vi "SPI_WRITE.vi"(0 "size(s) IN":i32, 1 "Data":u8) -> (6 "size(s)":i32, 7 "SDA":bool[](array[boolean]), 8 "SCL":bool[](array[boolean]), 9 "PFIWE":bool[](array[boolean]), 10 "ACK":i32)   [LabVIEW 2018]
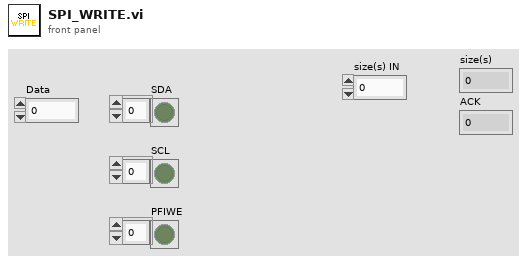
[diagram p1: front panel]
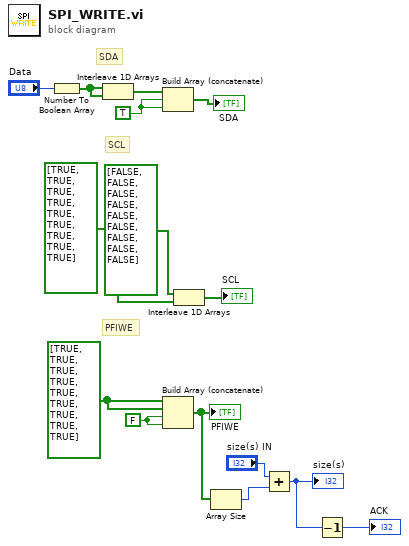
[diagram p0: block diagram]
diagram:
  w15 = FALSE
  w12 = TRUE
  w9 = bool[] [TRUE, TRUE, TRUE, TRUE, TRUE, TRUE, TRUE, TRUE, TRUE]
  # "PFIWE"
  # "SCL"
  # "SDA"
  n1 = Number To Boolean Array(number="Data") -> (Boolean array=w6:bool[])
  n2 = Interleave 1D Arrays(w6, w6) -> (w7:bool[])
  n3 = Build Array (concatenate)(w7, w12, w12) -> (→"SDA":bool[])
  n4 = Build Array (concatenate)(w9, w9, w15, w15) -> (w5:bool[])
  "PFIWE" <- w5
  n5 = Interleave 1D Arrays(bool[] [FALSE, FALSE, FALSE, FALSE, FALSE, FALSE, FALSE, FALSE, FALSE], bool[] [TRUE, TRUE, TRUE, TRUE, TRUE, TRUE, TRUE, TRUE, TRUE]) -> (→"SCL":bool[])
  n6 = Array Size(array=w5) -> (size(s)=w3:i32)
  n7 = Add(x="size(s) IN", y=w3) -> (x+y=w1:i32)
  "size(s)" <- w1
  n8 = Decrement(x=w1) -> (x-1=→"ACK":i32)
